vi "events_handler.vi"(1 "handler_index":dbl=9.0) -> ()   [LabVIEW 2018]
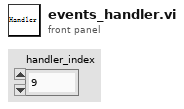
[diagram p1: front panel]
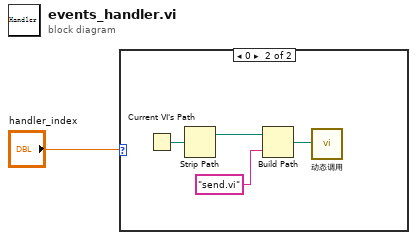
[diagram p0: block diagram]
diagram:
  n1 = case shown="0" "handler_index" {
    frame 9, Default {
    }
    frame 0 {
      n2 = Current VI's Path() -> (path=w3:path)
      n3 = Strip Path(path=w3) -> (stripped path=w4:path)  [unwired: 1 out]
      n4 = Build Path(base path=w4, name or relative path="send.vi" ("名称或相对路径")) -> (appended path=w5:path)
      n5 = call "动态调用.vi"("VI路径"=w5) -> ()  [unwired: 11 in]
    }
  }
